vi "Create Statement CSV.vi"(8 "Error In":errorcluster, 11 "Statement":T1) -> (0 "Error Out":errorcluster, 3 "CSV":string)   [LabVIEW 2017, in "Logger.lvlib"]
doc: "Converts a logging statement to a Comma Separated Values (CSV) line."
uses:
  Logger.lvlib
  Controls/Statement.ctl
  Controls/Tag.ctl
  <vilib>/dlg_ctls.llb/Space Constant.vi
  <vilib>/Utility/error.llb/Trim Whitespace.vi
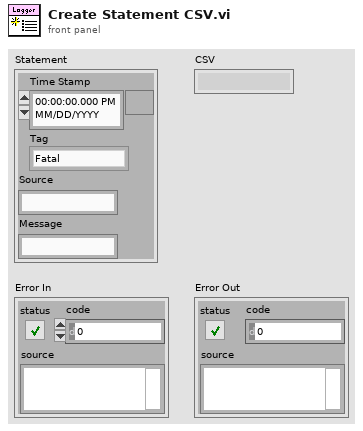
[diagram p1: front panel]
types:
  T1 = typedef "Logger.lvlib/Statement.ctl" = cluster{"Time Stamp":timestamp, "Tag":T2, "Source":string, "Message":string}
  T2 = typedef "Logger.lvlib/Tag.ctl" = enum16{"Fatal", "Error", "Warn", "Info", "Debug", "Trace"}
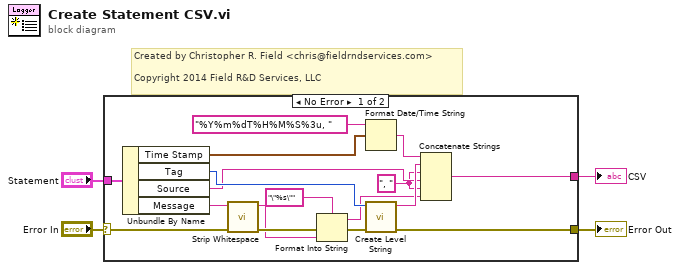
[diagram p0: block diagram]
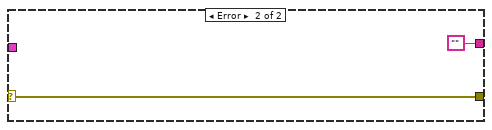
[diagram p2: hidden frame]
diagram:
  # "Created by Christopher R. Field <chris@fieldrndservices.com>\n\nCopyright 2014 Field R&D Services, LLC"
  n1 = case shown="No Error" "Error In" {
    selector: "Error In" -> [w11 w23]
    tunnel: "Statement" -> [w21 _]
    tunnel: [w13 w23] -> w2
    tunnel: [w12 ""] -> w1
    frame No Error {
      w14 = ", " ("string")
      n2 = Unbundle By Name(w21) -> ("Time Stamp"=w20:timestamp, "Tag"=w18:T2, "Source"=w15:string, "Message"=w9:string)
      n3 = call "Strip Whitespace.vi"("Error In"=w11, "Text"=w9) -> ("Error Out"=w10:errorcluster, "Stripped Text"=w6:string)  [unwired: 8 in]
      n4 = Format Into String(format string="\"%s\"", error in=w10, w6) -> (resulting string=w5:string, error out=w8:errorcluster)  [unwired: 1 in]
      n5 = Format Date/Time String(time format string (%c)="%Y%m%dT%H%M%S%3u, ", seconds (now)=w20) -> (date/time string=w17:string)  [unwired: 1 in]
      n6 = call "Create Level String.vi"("Error In"=w8, "Level"=w18) -> ("Error Out"=w13:errorcluster, "String"=w16:string)  [unwired: 8 in]
      n7 = Concatenate Strings(w17, w16, w14, w15, w14, w5) -> (w12:string)
    }
    frame Error {
    }
  }
  "Error Out" <- w2
  "CSV" <- w1
